vi "General - Split String.vi"(1 "Delimeter (;)":string=";", 2 "String":string) -> (0 "String Array":string[](array[string]))   [LabVIEW 2010]
doc: "Splits a single string into a string array by searching for a specific delimeter."
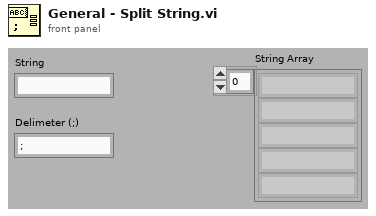
[diagram p1: front panel]
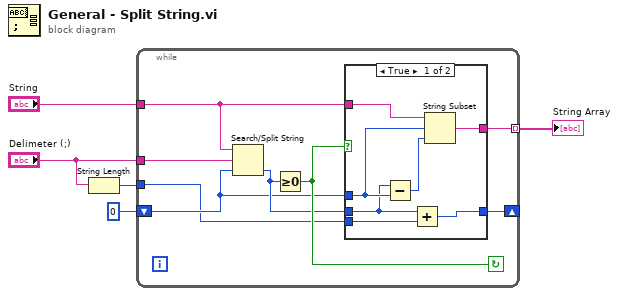
[diagram p0: block diagram]
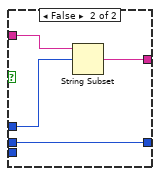
[diagram p2: hidden frame]
diagram:
  n1 = String Length(string="Delimeter (;)") -> (length=w4:i32)
  n2 = while {
    tunnel: [w12] -> w1 mode=indexing
    tunnel: "String" -> [w8]
    shift-right: [w10] -> _
    shift-left: 0 ("offset of match") -> [w9]
    tunnel: "Delimeter (;)" -> [w7]
    tunnel: w4 -> [w6]
    stop <- w13 continue-if-true
    n3 = Search/Split String(string=w8, search string/char (-)=w7, offset (0)=w9) -> (offset of match=w11:i32)  [unwired: 2 out]
    n4 = Greater Or Equal To 0?(x=w11) -> (x >= 0?=w13:bool)
    n5 = case shown="True" w13 {
      tunnel: [w20 w23] -> w12
      tunnel: w11 -> [w15 w21]
      tunnel: [w16 w21] -> w10
      tunnel: w9 -> [w17 w24]
      tunnel: w8 -> [w19 w22]
      tunnel: w6 -> [w14 _]
      frame True {
        n6 = Subtract(x=w15, y=w17) -> (x-y=w18:i32)
        n7 = Add(x=w15, y=w14) -> (x+y=w16:i32)
        n8 = String Subset(string=w19, offset (0)=w17, length (rest)=w18) -> (substring=w20:string)
      }
      frame False {
        n9 = String Subset(string=w22, offset (0)=w24) -> (substring=w23:string)  [unwired: 1 in]
      }
    }
  }
  "String Array" <- w1
